vi "Main.vi"() -> ()   [LabVIEW 2015]
uses:
  <vilib>/express/express analysis/Spectral/Block/exnSpectralBlock spectral measurements RMS poly.vi
  <vilib>/express/express analysis/Spectral/Block/exnSpectralBlock spectral measurements RMS WFM.vi
  <vilib>/imath/engines/lvmath2/RunTimeEngine/Managers/WorkSpace/UID Generator.vi
  <vilib>/imath/engines/lvmath2/RunTimeEngine/BuiltInFunctions/linramp/NIMS_linramp.vi
  <vilib>/imath/engines/lvmath2/RunTimeEngine/RunTimeType/NIMS_RunTimeType_From StrictType (excl LVString).vi
  <instcachedir>/0/NIMS_RunTimeType_From StrictType (excl LVString)_EB1C38A9BC5048DA9ABDA8F781E54D21.lvgen/NIMS_RunTimeType_From StrictType (excl LVString)_EB1C38A9BC5048DA9ABDA8F781E54D21_000.vi
  <vilib>/imath/engines/lvmath2/RunTimeEngine/LocalVariableDefStatement/MC_LocalVariableDefStatement_Display.vi
  <vilib>/imath/engines/lvmath2/RunTimeEngine/Managers/SymbolTable/Clear UID.vi
  <vilib>/imath/engines/lvmath2/RunTimeEngine/NodeEndStatement/NIMS_NodeEndStatement_Output.vi
  <instcachedir>/0/NIMS_NodeEndStatement_Output_53EC0D466D134D7ABD903AC30B43404B.lvgen/NIMS_NodeEndStatement_Output_53EC0D466D134D7ABD903AC30B43404B_005.vi
  <vilib>/imath/engines/lvmath2/RunTimeEngine/ErrorHandling/NIMS_Finalize Error.vi
  <vilib>/express/express analysis/Spectral/XNode/ExpressSpectralMeasurementsBlockNode.xnode
  <vilib>/imath/engines/lvmath2/RunTimeEngine/Managers/SymbolTable/NIMS_WorkSpace.lvlib
panel:
  in  "error in (no error)":errorcluster
  out "error out":errorcluster
  out "Waveform Graph":cluster{"f0":dbl, "df":dbl, "magnitude":dbl[]}(graph)={"f0"=0.0, "df"=5.0, "magnitude"=array[5000 elements]}
  in  "stop":bool
  in  "Time (s)":dbl=0.2
  in  "Rate":dbl=50000.0
  in  "Averages":i32=10
  out "?":waveform(dbl)(graph)={"t0"=timestamp(0 s since 1904-01-01), "dt"=2e-05, "Y"=array[10000 elements]}
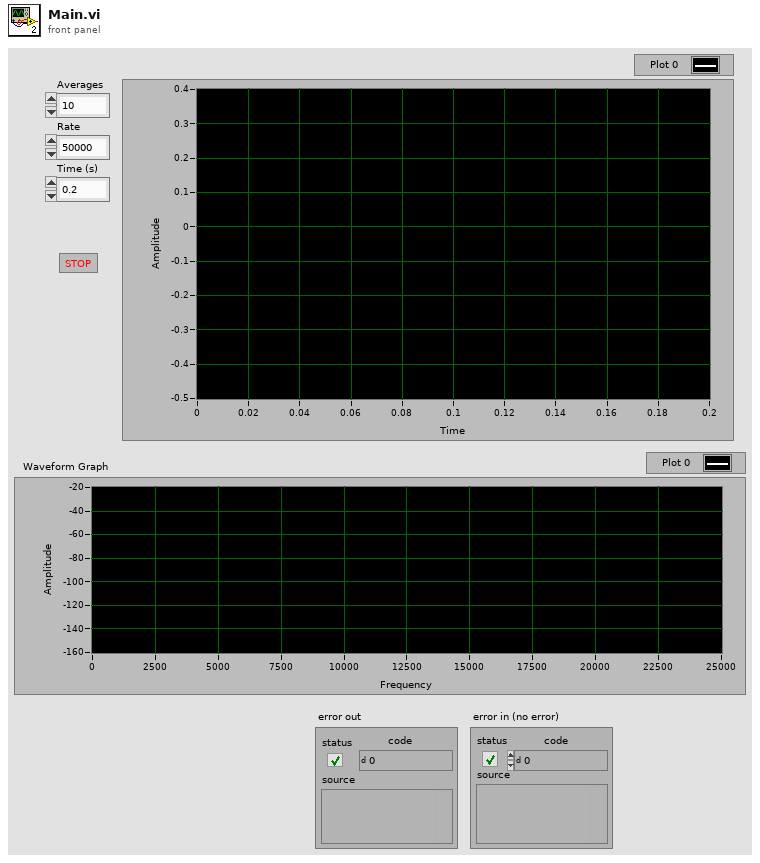
[diagram p1: front panel]
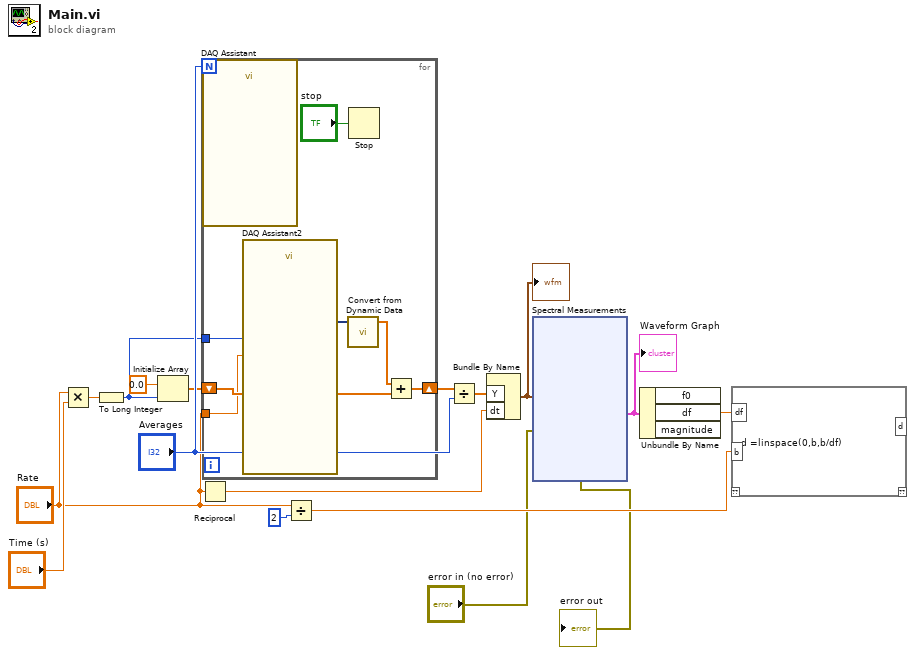
[diagram p0: block diagram]
diagram:
  n1 = Multiply(x="Rate", y="Time (s)") -> (x*y=w9:dbl)
  n2 = To Long Integer(number=w9) -> (32bit integer=w12:i32)
  n3 = Initialize Array(0.0, w12) -> (w15:dbl[])
  n4 = Reciprocal(x="Rate") -> (1/x=w8:dbl)
  n5 = for {
    N: "Averages" -> [_]
    shift-right: [w23] -> w14
    shift-left: w15 -> [w24]
    tunnel: w12 -> [w22]
    tunnel: "Rate" -> [w20]
    n6 = call "DAQ Assistant"() -> ()  [unwired: 18 in, 2 out]
    n7 = call "DAQ Assistant2"("rate"=w20, "number of samples"=w22) -> ("data"=w19:dynamicdata)  [unwired: 15 in, 2 out]
    n8 = call "Convert from Dynamic Data"("Dynamic Data Type"=w19) -> ("Array"=w18:dbl[])  [unwired: 3 in]
    n9 = Stop(stop? (T)="stop") -> ()
    n10 = Add(x=w18, y=w24) -> (x+y=w23:dbl[])
  }
  n11 = Divide(x="Rate", y=2) -> (x/y=w6:dbl)
  n12 = Divide(x=w14, y="Averages") -> (x/y=w10:dbl[])
  n13 = Bundle By Name("Y"=w10, "dt"=w8) -> (w11:waveform(dbl))  [unwired: 1 in]
  "?" <- w11
  n14 = xnode "Spectral Measurements"("Signals"=w11, "error in (no error)"="error in (no error)") -> ("FFT - (RMS)"=w3:cluster{"f0":dbl, "df":dbl, "magnitude":dbl[]}, "error out"=→"error out":errorcluster)  [unwired: 1 out]
  "Waveform Graph" <- w3
  n15 = Unbundle By Name(w3) -> ("df"=w4:dbl)  [unwired: 2 out]
  n16 = mathscript code="d =linspace(0,b,b/df)"("b"=w6, "df"=w4) -> ()  [unwired: 1 in, 2 out]
